vi "VI Server_Get ComboBox Selection.vi"(7 "Label":string, 8 "error in":errorcluster, 9 "Single Instance (T)":bool=TRUE, 11 "VI Server Cluster":T1) -> (0 "error out":errorcluster, 1 "CtrlRef":refnum<vi>, 2 "Selection":string, 3 "VI Server Cluster.DUP":T1, 4 "Value":string, 6 "Label.Text":string)   [LabVIEW 2020, in "VI Server Toolkit LV2013.lvlib"]
doc: "Returns selection of a Combo Box."
uses:
  VI Server Toolkit LV2013.lvlib
  VI Server_TypeDefs/VI Server_RefsCluster.ctl
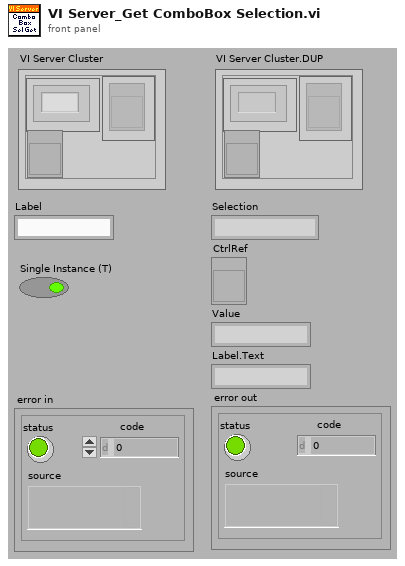
[diagram p1: front panel]
types:
  T1 = typedef "VI Server_RefsCluster.ctl" = cluster{"Labels":string[], "Refs":refnum<vi>[], "VI Ref":refnum<vi>}
  T2 = typedef "LVComboBoxStrsAndValuesArrayTypeDef.ctl" = cluster{"String":string, "Value":string}[]
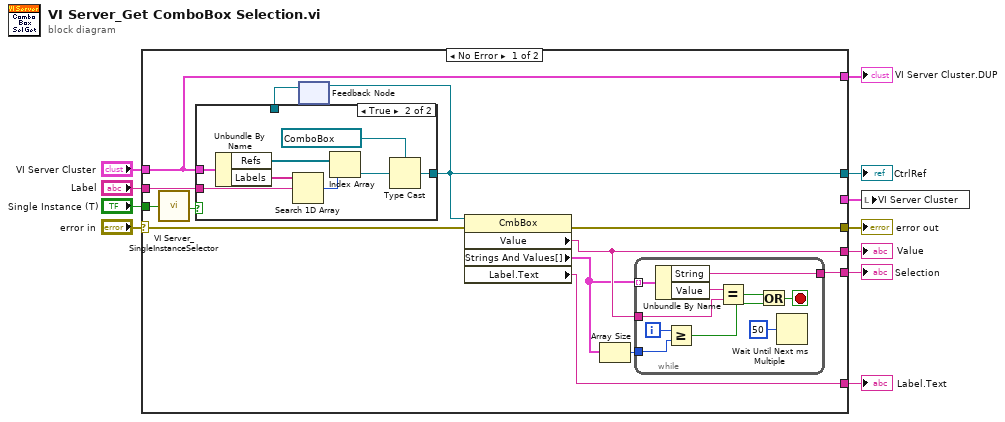
[diagram p0: block diagram]
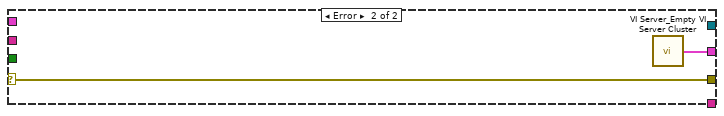
[diagram p3: hidden frame]
diagram:
  n1 = case shown="No Error" "error in" {
    selector: "error in" -> [w23 w45]
    tunnel: "Label" -> [w24 _]
    tunnel: "VI Server Cluster" -> [w16 _]
    tunnel: [w22 w45] -> w11
    tunnel: [w13 _] -> w5
    tunnel: [w20 _] -> w8
    tunnel: [w19 _] -> w7
    tunnel: [w21 _] -> w6
    tunnel: [w16 _] -> w3
    tunnel: "Single Instance (T)" -> [w14 _]
    tunnel: [_ w44] -> w1
    frame No Error {
      n2 = call "VI Server_SingleInstanceSelector.vi"("Single Instance (T)"=w14) -> ("Single Instance.OUT"=w15:bool)  [unwired: 6 in]
      n3 = feedback #1() -> (w12:refnum<vi>)  [unwired: 1 in]
      n4 = case shown="True" w15 {
        tunnel: w24 -> [_ w32]
        tunnel: [w25 w28] -> w13
        tunnel: w16 -> [_ w26]
        tunnel: w12 -> [w25 _]
        frame False {
        }
        frame True {
          n5 = Unbundle By Name(w26) -> ("Refs"=w30:refnum<vi>[], "Labels"=w33:string[])
          n6 = Search 1D Array(1D array=w33, element=w32) -> (index of element=w31:i32)  [unwired: 1 out]
          n7 = Index Array(array=w30, index=w31) -> (element=w29:refnum<vi>)
          n8 = Type Cast(type=refnum<vi> refnum ("PulceGen3.Trigger"), x=w29) -> (*(type *) &x=w28:refnum<vi>)
        }
      }
      n9 = feedback-in #1(w13) -> ()
      n10 = property class="CmbBox"(reference=w13, error in=w23) -> (error out=w22:errorcluster, "Value"=w19:string, "Strings And Values[]"=w18:T2, "Label.Text"=w21:string)  [unwired: 1 out]
      n11 = Array Size(array=w18) -> (size(s)=w17:i32)
      n12 = while {
        tunnel: w18 -> [w43] mode=indexing
        tunnel: [w42] -> w20
        tunnel: w19 -> [w40]
        tunnel: w17 -> [w36]
        i -> [w37]
        stop <- w34 stop-if-true
        n13 = Unbundle By Name(w43) -> ("String"=w42:string, "Value"=w41:string)
        n14 = Greater Or Equal?(x=w37, y=w36) -> (x >= y?=w35:bool)
        n15 = Equal?(x=w41, y=w40) -> (x = y?=w38:bool)
        n16 = Or(x=w38, y=w35) -> (x .or. y?=w34:bool)
        n17 = Wait Until Next ms Multiple(millisecond multiple=u32 50) -> ()  [unwired: 1 out]
      }
    }
    frame Error {
      n18 = call "VI Server_Empty VI Server Cluster.vi"() -> ("VI Server Cluster"=w44:T1)  [unwired: 7 in]
    }
  }
  "error out" <- w11
  "VI Server Cluster.DUP" <- w3
  "Selection" <- w8
  "Value" <- w7
  "Label.Text" <- w6
  "CtrlRef" <- w5
  n19 = local write "VI Server Cluster"(w1) -> ()
